vi "Tester.vi"() -> ()   [LabVIEW 2017]
panel:
  out "output array":u8[](array[numeric])
  in  "Tab Control":T1(tab)
  in  "Enable":bool
  in  "Timestep":u32
  in  "Port":u16=23456
  out "UDP timestep":u32(graph)
  in  "Send":bool
  in  "Port":u16=23456
  in  "unsigned byte array":u8[](array[numeric])=[2, 132, 1, 0, 1, 0, 1, 0, 1, 0]
  in  "Send":bool
  in  "index":i32=8 min=2 max=9
  # "uses port and data from single ping"
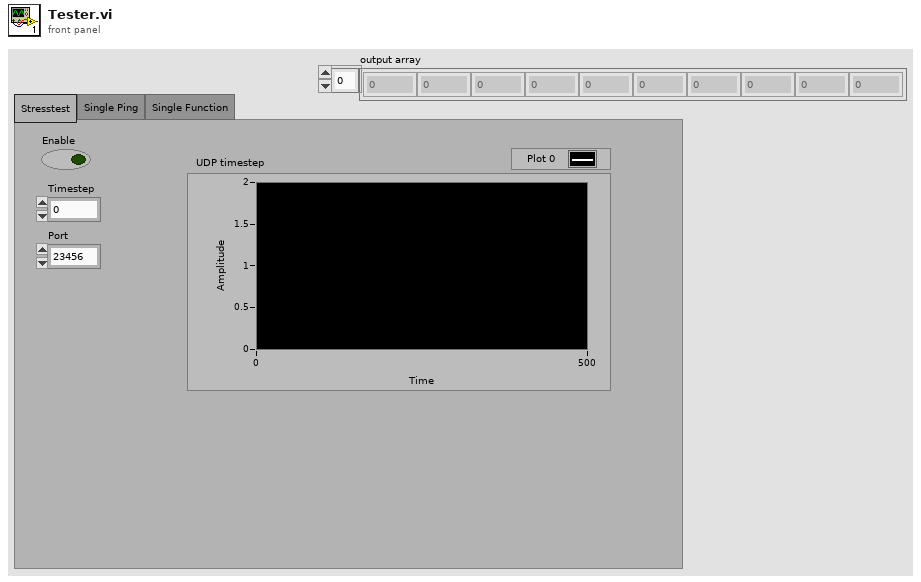
[diagram p1: front panel]
types:
  T1 = enum32{"Stresstest", "Single Ping", "Single Function"}
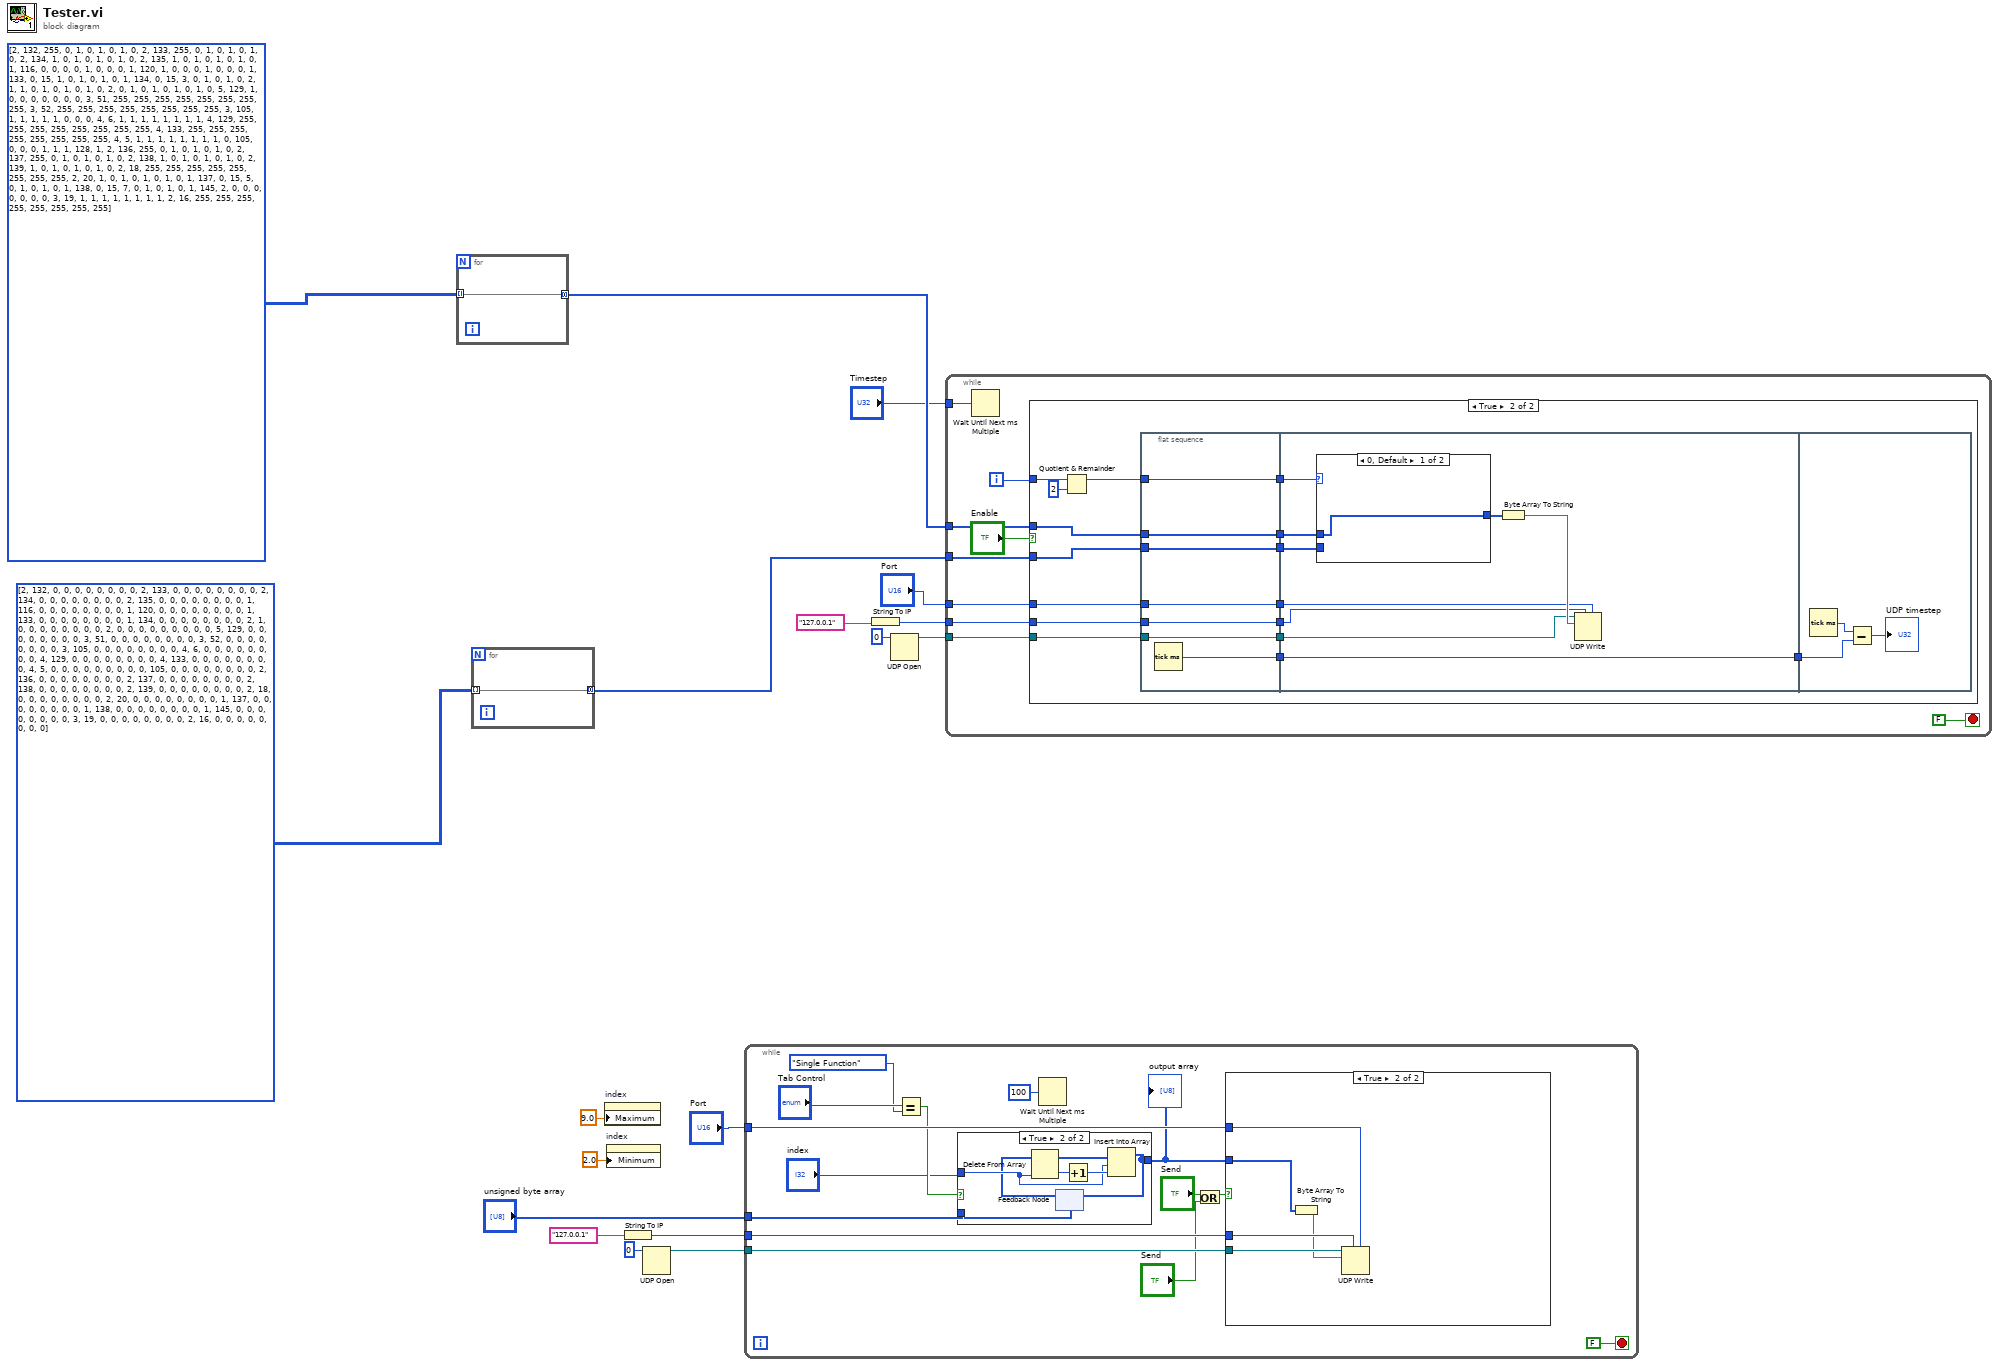
[diagram p0: block diagram]
diagram:
  n1 = for {
    tunnel: u8[][] [[2, 132, 255, 0, 1, 0, 1, 0, 1, 0], [2, 133, 255, 0, 1, 0, 1, 0, 1, 0], [2, 134, 1, 0, 1, 0, 1, 0, 1, 0], [2, 135, 1, 0, 1, 0, 1, 0, 1, 0], [1, 116, 0, 0, 0, 0, 1, 0, 0, 0], [1, 120, 1, 0, 0, 0, 1, 0, 0, 0], [1, 133, 0, 15, 1, 0, 1, 0, 1, 0], [1, 134, 0, 15, 3, 0, 1, 0, 1, 0], [2, 1, 1, 0, 1, 0, 1, 0, 1, 0], [2, 0, 1, 0, 1, 0, 1, 0, 1, 0], [5, 129, 1, 0, 0, 0, 0, 0, 0, 0], [3, 51, 255, 255, 255, 255, 255, 255, 255, 255], [3, 52, 255, 255, 255, 255, 255, 255, 255, 255], [3, 105, 1, 1, 1, 1, 1, 0, 0, 0], [4, 6, 1, 1, 1, 1, 1, 1, 1, 1], [4, 129, 255, 255, 255, 255, 255, 255, 255, 255], [4, 133, 255, 255, 255, 255, 255, 255, 255, 255], [4, 5, 1, 1, 1, 1, 1, 1, 1, 1], [0, 105, 0, 0, 0, 1, 1, 1, 128, 1], [2, 136, 255, 0, 1, 0, 1, 0, 1, 0], [2, 137, 255, 0, 1, 0, 1, 0, 1, 0], [2, 138, 1, 0, 1, 0, 1, 0, 1, 0], [2, 139, 1, 0, 1, 0, 1, 0, 1, 0], [2, 18, 255, 255, 255, 255, 255, 255, 255, 255], [2, 20, 1, 0, 1, 0, 1, 0, 1, 0], [1, 137, 0, 15, 5, 0, 1, 0, 1, 0], [1, 138, 0, 15, 7, 0, 1, 0, 1, 0], [1, 145, 2, 0, 0, 0, 0, 0, 0, 0], [3, 19, 1, 1, 1, 1, 1, 1, 1, 1], [2, 16, 255, 255, 255, 255, 255, 255, 255, 255]] ("stresstest1") -> [w19] mode=indexing
    tunnel: [w19] -> w17 mode=concatenating
  }
  n2 = for {
    tunnel: u8[][] [[2, 132, 0, 0, 0, 0, 0, 0, 0, 0], [2, 133, 0, 0, 0, 0, 0, 0, 0, 0], [2, 134, 0, 0, 0, 0, 0, 0, 0, 0], [2, 135, 0, 0, 0, 0, 0, 0, 0, 0], [1, 116, 0, 0, 0, 0, 0, 0, 0, 0], [1, 120, 0, 0, 0, 0, 0, 0, 0, 0], [1, 133, 0, 0, 0, 0, 0, 0, 0, 0], [1, 134, 0, 0, 0, 0, 0, 0, 0, 0], [2, 1, 0, 0, 0, 0, 0, 0, 0, 0], [2, 0, 0, 0, 0, 0, 0, 0, 0, 0], [5, 129, 0, 0, 0, 0, 0, 0, 0, 0], [3, 51, 0, 0, 0, 0, 0, 0, 0, 0], [3, 52, 0, 0, 0, 0, 0, 0, 0, 0], [3, 105, 0, 0, 0, 0, 0, 0, 0, 0], [4, 6, 0, 0, 0, 0, 0, 0, 0, 0], [4, 129, 0, 0, 0, 0, 0, 0, 0, 0], [4, 133, 0, 0, 0, 0, 0, 0, 0, 0], [4, 5, 0, 0, 0, 0, 0, 0, 0, 0], [0, 105, 0, 0, 0, 0, 0, 0, 0, 0], [2, 136, 0, 0, 0, 0, 0, 0, 0, 0], [2, 137, 0, 0, 0, 0, 0, 0, 0, 0], [2, 138, 0, 0, 0, 0, 0, 0, 0, 0], [2, 139, 0, 0, 0, 0, 0, 0, 0, 0], [2, 18, 0, 0, 0, 0, 0, 0, 0, 0], [2, 20, 0, 0, 0, 0, 0, 0, 0, 0], [1, 137, 0, 0, 0, 0, 0, 0, 0, 0], [1, 138, 0, 0, 0, 0, 0, 0, 0, 0], [1, 145, 0, 0, 0, 0, 0, 0, 0, 0], [3, 19, 0, 0, 0, 0, 0, 0, 0, 0], [2, 16, 0, 0, 0, 0, 0, 0, 0, 0]] ("stresstest2") -> [w20] mode=indexing
    tunnel: [w20] -> w15 mode=concatenating
  }
  n3 = property on="index" class="DigNum (strict)"("Maximum"=9.0 ("Data Entry Limits:Maximum")) -> ()  [unwired: 2 in, 2 out]
  n4 = property on="index" class="DigNum (strict)"("Minimum"=2.0 ("Data Entry Limits:Minimum")) -> ()  [unwired: 2 in, 2 out]
  n5 = String To IP(1:"127.0.0.1" ("ip")) -> (0:w5:u32)
  n6 = UDP Open(11:u16 0 ("port")) -> (port=w6:refnum<k16>)  [unwired: 4 in, 2 out]
  n7 = while {
    tunnel: w6 -> [w32]
    tunnel: w5 -> [w31]
    tunnel: "Port" -> [w30]
    tunnel: "unsigned byte array" -> [w29]
    stop <- FALSE stop-if-true
    n8 = Equal?(x="Tab Control", y=T1."Single Function") -> (x = y?=w22:bool)
    n9 = case shown="True" w22 {
      tunnel: w29 -> [w35 w42]
      tunnel: "index" -> [_ w39]
      tunnel: [w35 w37] -> w28
      frame False {
      }
      frame True {
        n10 = feedback #1(w42) -> (w38:u8[])
        n11 = Delete From Array(array=w38, index=w39) -> (deleted portion=w41:u8, array with subset deleted=w36:u8[])  [unwired: 1 in]
        n12 = Increment(x=w41) -> (x+1=w40:u8)
        n13 = Insert Into Array(array=w36, index=w39, new element=w40) -> (w37:u8[])
        n14 = feedback-in #1(w37) -> ()
      }
    }
    "output array" <- w28
    n15 = Wait Until Next ms Multiple(millisecond multiple=u32 100) -> ()  [unwired: 1 out]
    n16 = Or(x="Send", y="Send") -> (x .or. y?=w26:bool)
    n17 = case shown="True" w26 {
      tunnel: w32 -> [_ w47]
      tunnel: w31 -> [_ w46]
      tunnel: w30 -> [_ w45]
      tunnel: w28 -> [_ w44]
      frame False {
      }
      frame True {
        n18 = Byte Array To String(unsigned byte array=w44) -> (string=w43:string)
        n19 = UDP Write(address=w46, port or service name=w45, connection ID=w47, data in=w43) -> ()  [unwired: 2 in, 2 out]
      }
    }
  }
  n20 = String To IP(1:"127.0.0.1" ("ip")) -> (0:w12:u32)
  n21 = UDP Open(11:u16 0 ("port")) -> (port=w14:refnum<k16>)  [unwired: 4 in, 2 out]
  n22 = while {
    tunnel: w15 -> [w54]
    tunnel: w17 -> [w53]
    tunnel: "Timestep" -> [w51]
    tunnel: w14 -> [w50]
    tunnel: "Port" -> [w49]
    tunnel: w12 -> [w48]
    i -> [w56]
    stop <- FALSE stop-if-true
    n23 = Wait Until Next ms Multiple(millisecond multiple=w51) -> ()  [unwired: 1 out]
    n24 = case shown="True" "Enable" {
      tunnel: w56 -> [_ w69]
      tunnel: w54 -> [_ w66]
      tunnel: w53 -> [_ w65]
      tunnel: w50 -> [_ w61]
      tunnel: w49 -> [_ w59]
      tunnel: w48 -> [_ w57]
      frame False {
      }
      frame True {
        n25 = Quotient & Remainder(x=w69, y=2) -> (x-y*floor(x/y)=w67:i32)  [unwired: 1 out]
        n26 = flat-sequence {
          tunnel: [w79] -> w72
          tunnel: w67 -> [w79]
          tunnel: [w77] -> w71
          tunnel: [w78] -> w70
          tunnel: w66 -> [w78]
          tunnel: w65 -> [w77]
          tunnel: [w76] -> w63
          tunnel: [w75] -> w62
          tunnel: w61 -> [w75]
          tunnel: [w74] -> w60
          tunnel: w59 -> [w74]
          tunnel: [w73] -> w58
          tunnel: w57 -> [w73]
          tunnel: w72 -> [w88]
          tunnel: w71 -> [w87]
          tunnel: w70 -> [w86]
          tunnel: [w84] -> w64
          tunnel: w63 -> [w84]
          tunnel: w62 -> [w82]
          tunnel: w60 -> [w81]
          tunnel: w58 -> [w80]
          tunnel: w64 -> [w92]
          frame #0 {
            n27 = Tick Count (ms)() -> (millisecond timer value=w76:u32)
          }
          frame #1 {
            n28 = case shown="0, Default" w88 {
              tunnel: [w89 w90] -> w85
              tunnel: w87 -> [w89 _]
              tunnel: w86 -> [_ w90]
              frame 0, Default {
              }
              frame 1 {
              }
            }
            n29 = Byte Array To String(unsigned byte array=w85) -> (string=w83:string)
            n30 = UDP Write(address=w80, port or service name=w81, connection ID=w82, data in=w83) -> ()  [unwired: 2 in, 2 out]
          }
          frame #2 {
            n31 = Tick Count (ms)() -> (millisecond timer value=w93:u32)
            n32 = Subtract(x=w93, y=w92) -> (x-y=→"UDP timestep":u32)
          }
        }
      }
    }
  }
